vi "Copy Template Code.vi"(8 "error in (no error)":errorcluster) -> (0 "error out":errorcluster)   [LabVIEW 2016, in "SLL Class DVR API Generator.lvlib"]
uses:
  SLL Class DVR API Generator.lvlib
  Template/__DVR API Template.vi
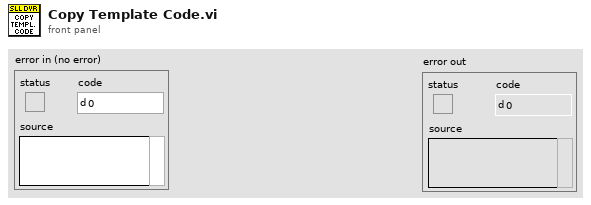
[diagram p1: front panel]
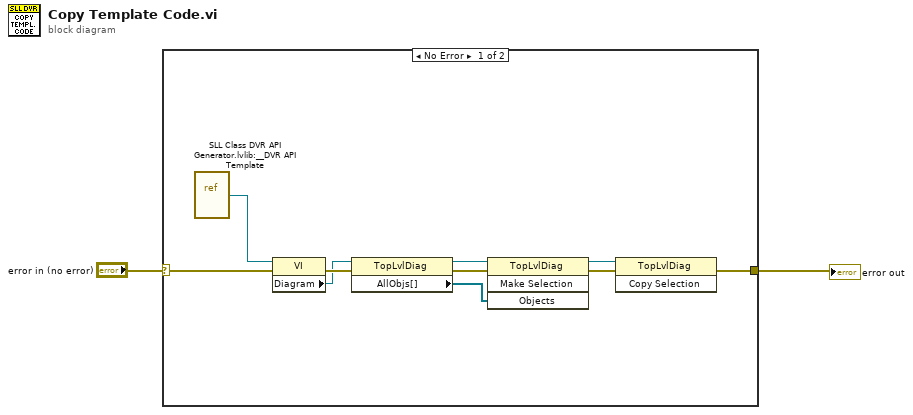
[diagram p0: block diagram]
diagram:
  n1 = case shown="No Error" "error in (no error)" {
    selector: "error in (no error)" -> [w4 w13]
    tunnel: [w6 w13] -> w1
    frame No Error {
      n2 = vi-ref "SLL Class DVR API Generator.lvlib:__DVR API Template.vi"() -> (w3:refnum<vi>)
      n3 = property class="VI"(reference=w3, error in=w4) -> (error out=w12:errorcluster, "Diagram"=w10:refnum<vi>)  [unwired: 1 out]
      n4 = property class="TopLvlDiag"(reference=w10, error in=w12) -> (reference out=w8:refnum<vi>, error out=w11:errorcluster, "AllObjs[]"=w7:refnum<vi>[])
      n5 = invoke class="TopLvlDiag" method="Make Selection"(reference=w8, error in=w11, "Objects"=w7) -> (reference out=w5:refnum<vi>, error out=w9:errorcluster)  [unwired: 1 in, 2 out]
      n6 = invoke class="TopLvlDiag" method="Copy Selection"(reference=w5, error in=w9) -> (error out=w6:errorcluster)  [unwired: 1 in, 2 out]
    }
    frame Error {
    }
  }
  "error out" <- w1
